vi "HISTORY_RECORDER_EPICSold.vi"() -> ()   [LabVIEW 2015]
uses:
  <vilib>/Platform/TimedLoop/XDataNode/timing_clust.ctl
  <vilib>/Platform/TimedLoop/XDataNode/nitl_modes.ctl
  <vilib>/Platform/TimedLoop/XDataNode/wakeup.ctl
  <vilib>/Utility/config.llb/Read Key (String).vi
  <vilib>/Utility/config.llb/Read Key (Path).vi
  <userlib>/caLab/Private/Get_PV-1D.vi
  <vilib>/platform/TimedLoop/XDataNode/XDataNode.xnode
  <vilib>/Utility/config.llb/NI_LVConfig.lvlib
  <vilib>/Platform/TimedLoop/XDataNode/XDNodeRunTimeDep.lvlib
panel:
  out "Number of Columns":u32
  out "file path 2":path=path "S:/"
  out "PV name array":string[](array[string])
  out "spreadsheet string":string
  out "file path":path=path "S:/"
  out "current time":timestamp
  out "PV Array":dbl[][](array[numeric])
  out "PV Names (dup)":string[](array[string])
  in  "JPEG":path
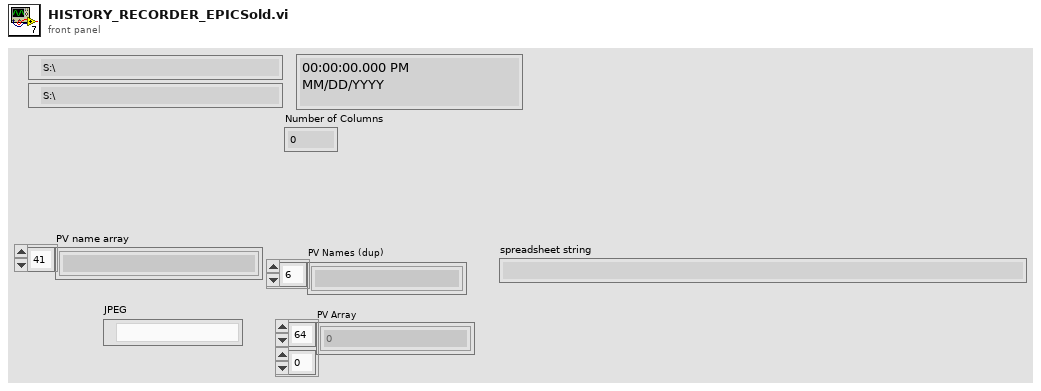
[diagram p1: front panel]
types:
  T1 = typedef "NI_LVConfig.lvlib/Config Data RefNum.ctl" = refnum<k1>
  T2 = typedef "XDNodeRunTimeDep.lvlib/timing_clust.ctl" = cluster{"Expected End [f-1]":u64, "Actual End [f-1]":u64, "Finished Late? [f-1]":bool, "Expected End [i-1]":u64, "Actual End [i-1]":u64, "Finished Late? [i-1]":bool, "Expected Start [i]":u64, "Actual Start [i]":u64, "Expected Start [f]":u64, "Actual Start [f]":u64, "Source Name":string, "Structure Name":string, "Period":i64, "Deadline":i64, "Offset":i64, "Start":i64, "Priority":i32, "Timeout":i32, "Mode":T3, "Wakeup Reason":T4, "Error":errorcluster, "Source Type":string, "Secondary Source Type":string, "Global End Time":u64, "Global Start Time":u64, "Frame Duration":u64, "Iteration Duration":u64, "Assigned CPU":i32, "I/O Scan Engine Mode":u32}
  T3 = typedef "XDNodeRunTimeDep.lvlib/nitl_modes.ctl" = enum32{"No Change", "Process missed periods, maintain original phase", "Discard missed periods, maintain original phase", "Process missed periods, ignore original phase", "Discard missed periods, ignore original phase"}
  T4 = typedef "XDNodeRunTimeDep.lvlib/wakeup.ctl" = enum32{"Normal", "Aborted", "Asynchronous wakeup", "Timing source error", "Timed loop error", "Timeout"}
  T5 = enum16{"open", "replace", "create", "open or create", "replace or create", "replace or create with confirmation"}
  T6 = typedef "imagedata.ctl" = cluster{"image type":i32, "image depth":i32, "image":u8[], "mask":u8[], "colors":u32[], "Rectangle":cluster{"left":i16, "top":i16, "right":i16, "bottom":i16}}
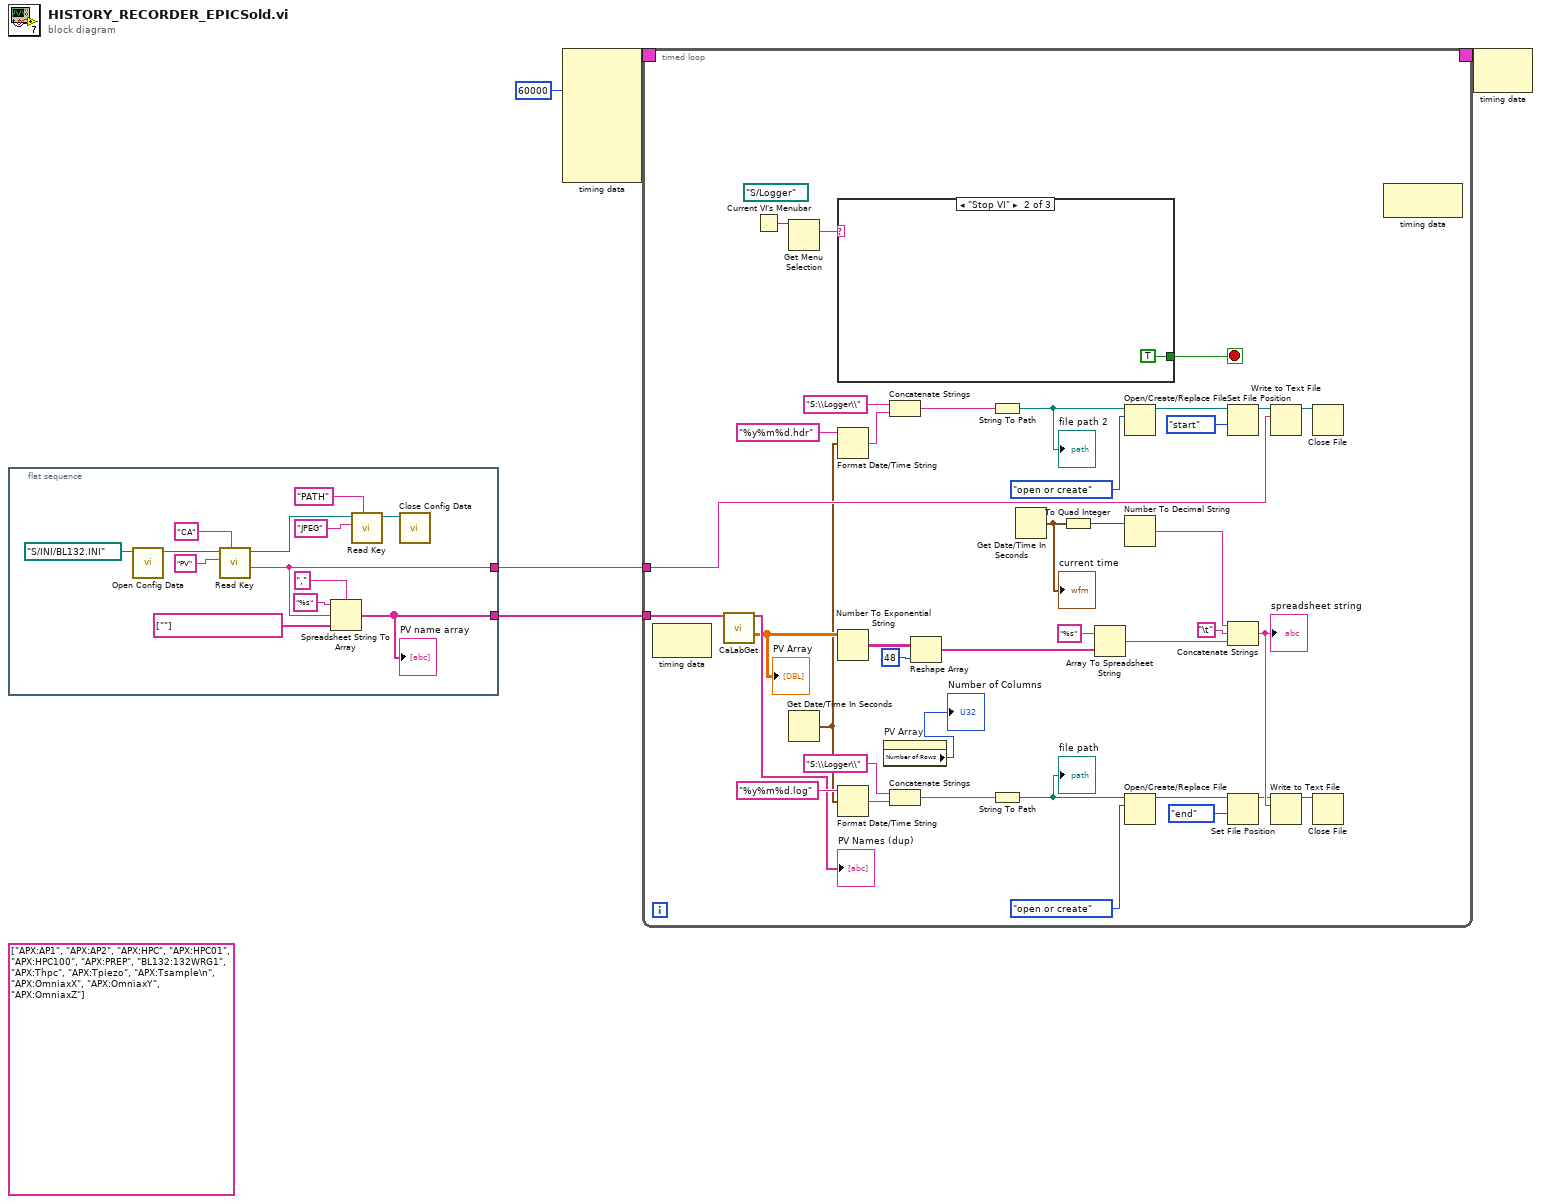
[diagram p0: block diagram]
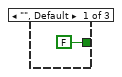
[diagram p2: hidden frame]
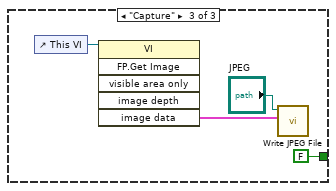
[diagram p3: hidden frame]
diagram:
  (unwired) string[] ["APX:AP1", "APX:AP2", "APX:HPC", "APX:HPC01", "APX:HPC100", "APX:PREP", "BL132:132WRG1", "APX:Thpc", "APX:Tpiezo", "APX:Tsample\n", "APX:OmniaxX", "APX:OmniaxY", "APX:OmniaxZ"]
  n1 = flat-sequence {
    tunnel: [w8] -> w2
    tunnel: [w6] -> w1
    frame #0 {
      n2 = call <vilib>:"Open Config Data.vi"("configuration file path"=path "S:/INI/BL132.INI") -> ("refnum"=w14:T1)  [unwired: 8 in, 2 out]
      n3 = call-poly <vilib>:"Read Key.vi"("section"="CA", "key"="PV", "refnum"=w14) -> ("value"=w6:string, "refnum out"=w9:T1)  [unwired: 5 in, 2 out]
      n4 = Spreadsheet String To Array(delimiter (Tab)=",", format string="%s", spreadsheet string=w6, array type (2D Dbl)=string[] [""] ("Strings []")) -> (array=w8:string[])
      "PV name array" <- w8
      n5 = call-poly <vilib>:"Read Key.vi"("section"="PATH" ("key"), "key"="JPEG" ("section"), "refnum"=w9) -> ("refnum out"=w18:T1)  [unwired: 5 in, 3 out]
      n6 = call <vilib>:"Close Config Data.vi"("refnum"=w18) -> ()  [unwired: 9 in, 2 out]
    }
  }
  n7 = node-c288(i64 60000 ("Period")) -> (w5:T2)  [unwired: 6 in]
  n8 = timed-loop {
    timing: w5 -> [_]
    timing-out: [_] -> w4
    tunnel: w2 -> [w38]
    tunnel: w1 -> [w24]
    stop <- w55 stop-if-true
    (unwired) path "S:/Logger" ("configuration file path")
    n9 = node-c288() -> ()  [unwired: 1 in, 1 out]
    n10 = call-poly <userlib>:"CaLabGet.vi"("PV Names"=w38) -> ("PV Names (dup)"=→"PV Names (dup)":string[], "Value Array (number)"=w36:dbl[][])  [unwired: 8 in, 5 out]
    "PV Array" <- w36
    n11 = Current VI's Menubar() -> (w57:refnum<k9>)
    n12 = Get Menu Selection(0:w57) -> (6:w56:string)  [unwired: 3 in, 4 out]
    n13 = Get Date/Time In Seconds() -> (seconds since 1Jan1904=w23:timestamp)
    n14 = case shown="\"Stop VI\"" w56 {
      tunnel: [FALSE TRUE FALSE] -> w55
      frame "", Default {
      }
      frame "Stop VI" {
      }
      frame "Capture" {
        n15 = control-ref of="This VI"() -> (w62:refnum<vi>)
        n16 = invoke class="VI" method="FP.Get Image"(reference=w62) -> ("image data"=w61:T6)  [unwired: 5 in, 5 out]
        n17 = call <vilib>:"Write JPEG File.vi"("image data"=w61, "path to JPEG file"="JPEG") -> ()  [unwired: 8 in, 2 out]
      }
    }
    n18 = Format Date/Time String(time format string (%c)="%y%m%d.hdr", seconds (now)=w23) -> (date/time string=w27:string)  [unwired: 1 in]
    n19 = Number To Exponential String(number=w36) -> (E-format string=w53:string[][])  [unwired: 3 in]
    n20 = Format Date/Time String(time format string (%c)="%y%m%d.log", seconds (now)=w23) -> (date/time string=w40:string)  [unwired: 1 in]
    n21 = property on="PV Array" class="Arr (strict)"() -> ("Number of Rows"=→"Number of Columns":u32)  [unwired: 2 in, 2 out]
    n22 = Concatenate Strings("S:\\Logger\\", w27) -> (w28:string)
    n23 = Concatenate Strings("S:\\Logger\\", w40) -> (w39:string)
    n24 = Reshape Array(w53, 48 ("dimension size")) -> (w51:string[])
    n25 = String To Path(string=w28) -> (path=w29:path)
    "file path 2" <- w29
    n26 = String To Path(string=w39) -> (path=w43:path)
    "file path" <- w43
    n27 = Get Date/Time In Seconds() -> (seconds since 1Jan1904=w54:timestamp)
    "current time" <- w54
    n28 = To Quad Integer(1:w54) -> (0:w48:i64)
    n29 = Array To Spreadsheet String(array=w51, 3:"%s" ("format string")) -> (spreadsheet string=w49:string)  [unwired: 1 in]
    n30 = Open/Create/Replace File(file path (use dialog)=w29, operation (0:open)=T5."open or create" ("operation (0:open) 2")) -> (refnum out=w21:refnum<file>)  [unwired: 4 in, 2 out]
    n31 = Number To Decimal String(number=w48) -> (decimal integer string=w46:string)  [unwired: 1 in]
    n32 = Open/Create/Replace File(file path (use dialog)=w43, operation (0:open)=T5."open or create") -> (refnum out=w33:refnum<file>)  [unwired: 4 in, 2 out]
    n33 = Set File Position(refnum=w21, from (0:start)=enum16{"start", "end", "current"}."start") -> (refnum out=w20:refnum<file>)  [unwired: 2 in, 1 out]
    n34 = Concatenate Strings(w46, "\t", w49) -> (w45:string)
    "spreadsheet string" <- w45
    n35 = Set File Position(refnum=w33, from (0:start)=enum16{"start", "end", "current"}."end") -> (refnum out=w32:refnum<file>)  [unwired: 2 in, 1 out]
    n36 = Write to Text File(file (use dialog)=w20, text=w24) -> (refnum out=w30:refnum<file>)  [unwired: 2 in, 2 out]
    n37 = Write to Text File(file (use dialog)=w32, text=w45) -> (refnum out=w44:refnum<file>)  [unwired: 2 in, 2 out]
    n38 = Close File(refnum=w30) -> ()  [unwired: 1 in, 2 out]
    n39 = Close File(refnum=w44) -> ()  [unwired: 1 in, 2 out]
    n40 = node-c288() -> ()  [unwired: 1 in, 1 out]
  }
  n41 = node-c288(w4) -> ()  [unwired: 1 out]
